vi "Read license file.vi"(8 "error in (no error)":errorcluster, 11 "file path":path) -> (0 "error out":errorcluster, 2 "MD5 Message Digest":string, 3 "file path out":path)   [LabVIEW 2016]
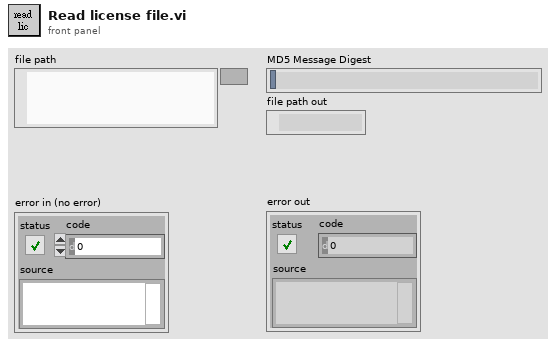
[diagram p1: front panel]
types:
  T1 = enum16{"open", "replace", "create", "open or create", "replace or create", "replace or create with confirmation"}
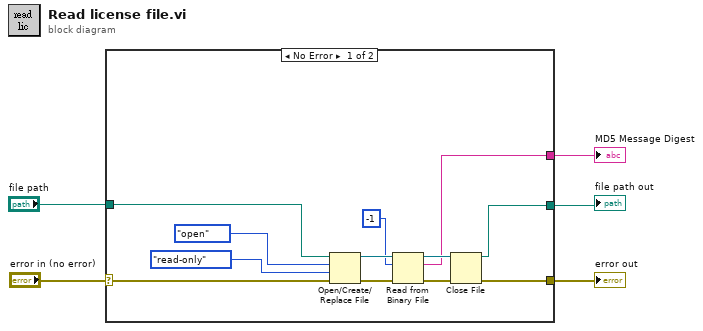
[diagram p0: block diagram]
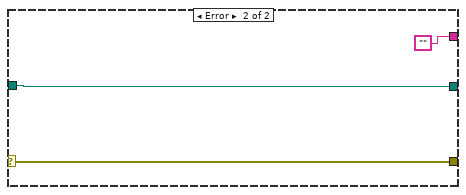
[diagram p2: hidden frame]
diagram:
  n1 = case shown="No Error" "error in (no error)" {
    selector: "error in (no error)" -> [w9 w20]
    tunnel: "file path" -> [w17 w18]
    tunnel: [w8 w20] -> w3
    tunnel: [w7 ""] -> w2
    tunnel: [w6 w18] -> w1
    frame No Error {
      n2 = Open/Create/Replace File(file path (use dialog)=w17, error in=w9, operation (0:open)=T1."open", access (0:read/write)=enum16{"read/write", "read-only", "write-only"}."read-only") -> (refnum out=w14:refnum<file>, error out=w13:errorcluster)  [unwired: 2 in, 1 out]
      n3 = Read from Binary File(8:w13, 10:-1 ("count (1)"), 11:w14) -> (0:w12:errorcluster, 2:w7:string, 3:w11:refnum<file>)  [unwired: 3 in, 1 out]
      n4 = Close File(refnum=w11, error in=w12) -> (path=w6:path, error out=w8:errorcluster)
    }
    frame Error {
    }
  }
  "error out" <- w3
  "MD5 Message Digest" <- w2
  "file path out" <- w1
